vi "To String (Boolean).vi"(8 "error in (no error)":errorcluster, 11 "JSON Value in":variant) -> (0 "error out":errorcluster, 3 "String":string)   [LabVIEW 2017, in "Advanced Variant Tools.lvlib"]
uses:
  Advanced Variant Tools.lvlib
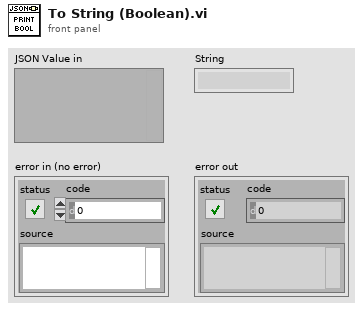
[diagram p1: front panel]
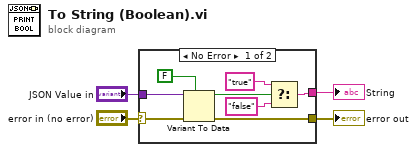
[diagram p0: block diagram]
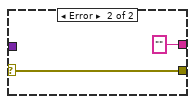
[diagram p2: hidden frame]
diagram:
  n1 = case shown="No Error" "error in (no error)" {
    selector: "error in (no error)" -> [w7 w13]
    tunnel: "JSON Value in" -> [w12 _]
    tunnel: [w9 "" ("f")] -> w3
    tunnel: [w6 w13] -> w1
    frame No Error {
      n2 = Variant To Data(error in=w7, type=FALSE, Variant=w12) -> (data=w5:bool, error out=w6:errorcluster)
      n3 = Select(t="true" ("String"), s=w5, f="false") -> (s? t:f=w9:string)
    }
    frame Error {
    }
  }
  "String" <- w3
  "error out" <- w1
